vi "Levels (1 Ch).vi"(8 "error in (no error)":errorcluster, 11 "Waveform":waveform(sgl)) -> (0 "error out":errorcluster, 1 "Pk-Pk":sgl, 2 "Peak":sgl, 3 "Crest Factor":sgl, 4 "Derived Peak":sgl, 5 "RMS":sgl)   [LabVIEW 2017, in "VibrationAnalysisFunctions.lvlib"]
doc: "Calculates true peak and true pk-pk in EU."
uses:
  <vilib>/addons/InsightCM/Utilities/Analysis/Vibration/VibrationAnalysisFunctions.lvlib
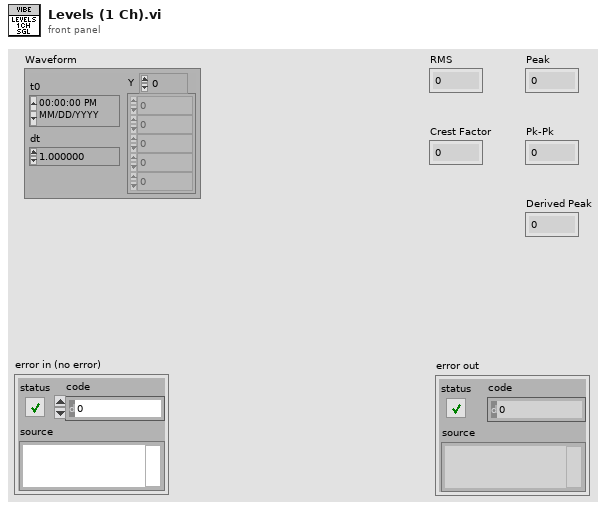
[diagram p1: front panel]
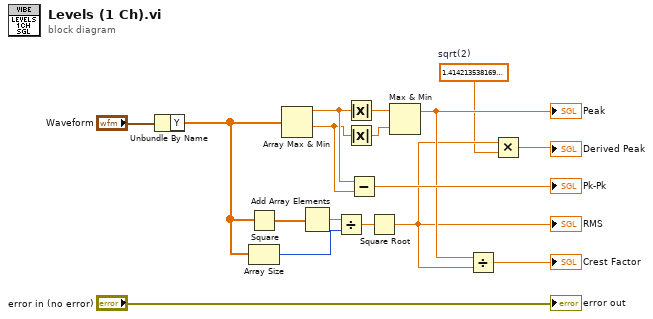
[diagram p0: block diagram]
diagram:
  w1 = sgl 1.4142135  # sqrt(2)
  n1 = Unbundle By Name("Waveform") -> ("Y"=w9:sgl[])
  n2 = Square(x=w9) -> (x^2=w10:sgl[])
  n3 = Array Size(array=w9) -> (size(s)=w7:i32)
  n4 = Array Max & Min(array=w9) -> (max value=w14:sgl, min value=w13:sgl)  [unwired: 2 out]
  n5 = Add Array Elements(numeric array=w10) -> (sum=w8:sgl)
  n6 = Divide(x=w8, y=w7) -> (x/y=w6:sgl)
  n7 = Absolute Value(x=w14) -> (abs(x)=w16:sgl)
  n8 = Absolute Value(x=w13) -> (abs(x)=w15:sgl)
  n9 = Subtract(x=w14, y=w13) -> (x-y=→"Pk-Pk":sgl)
  n10 = Square Root(x=w6) -> (sqrt(x)=w3:sgl)
  "RMS" <- w3
  n11 = Max & Min(x=w16, y=w15) -> (max(x,y)=w5:sgl)  [unwired: 1 out]
  "Peak" <- w5
  n12 = Divide(x=w5, y=w3) -> (x/y=→"Crest Factor":sgl)
  n13 = Multiply(x=w3, y=w1) -> (x*y=→"Derived Peak":sgl)
  "error out" <- "error in (no error)"
